vi "PIM Convert 1.1 to 1.2.vi"(0 "PIM 1.1 Test Parameters":T8={"PIM Test Stimulus"={"C1 Pwr dBm"=0.0, "C2 Pwr dBm"=0.0, "Power Units"=enum."dBm", "Meas Type"=enum."Band Edges", "C1 Fixed MHz"=0.0, "C2 Fixed MHz"=0.0, "Swept Freq Step"=0}, "Measure"={"IM Order"=0, "Direction"=0, "Averaging"=1, "ALC ON?"=TRUE, "Peak Hold?"=TRUE, "Peak last N"=1, "Ref Level dBm"=-100.0, "Ref Units"=enum."dBm", "Num Samples"=1, "Sample units"=enum."Sample(s)", "Update Rate (s)"=0.0}, "Display"={"Power Scale"={"yRange_min"=-160, "yRange_max"=-60}, "xRange_span"=0}, "Datasheets"=[]} {"Display"."xRange_span" min=5 step=1; "Display"."Power Scale"."yRange_max" min=-200 max=0 step=1; "Display"."Power Scale"."yRange_min" min=-200 max=0 step=1; "Measure"."Update Rate (s)" min=-200.0 max=0.0 step=0.2 format="%.1f"; "Measure"."Num Samples" min=1 max=5000 step=1; "Measure"."Averaging" items=["None", "Minimum", "Normal", "High", "Maximum"]; "Measure"."Ref Level dBm" min=-200.0 max=0.0 step=0.2 format="%.1f"; "Measure"."Peak last N" min=1 max=5000 step=1; "Measure"."Direction" items=["Reverse", "Forward", "Auxiliary"]; "Measure"."IM Order" items=["3rd", "5th", "7th", "9th", "11th", "13th", "15th", "17th", "19th", "21st", "23rd", "25th", "27th", "29th", "31st", "33rd"]; "PIM Test Stimulus"."C2 Fixed MHz" min=-200.0 max=0.0 step=0.2 format="%.1f"; "PIM Test Stimulus"."C1 Fixed MHz" min=-200.0 max=0.0 step=0.2 format="%.1f"; "PIM Test Stimulus"."Swept Freq Step" items=[".2", ".4", "1.0", "2.0"]}) -> (1 "Datasheets":T7, 2 "PIM 1.2 Test Parameters":T1={"Stimulus"={"C1 Pwr dBm"=0.0, "C2 Pwr dBm"=0.0, "Power Units"=enum."dBm", "Meas Type"=enum."Fixed Pair", "C1 Fixed MHz"=0.0, "C2 Fixed MHz"=0.0, "Swept Freq Step"=0}, "Measure"={"IM Order"=0, "Direction"=0, "Averaging"=0, "ALC ON?"=FALSE, "Peak Hold?"=FALSE, "Peak last N"=0, "Ref Level dBm"=0.0, "Ref Units"=enum."dBm", "Num Samples"=0, "Sample units"=enum."Sample(s)", "Update Rate (s)"=0.0}, "Display"={"Power Scale"={"yRange_min"=0, "yRange_max"=0}, "xRange_span"=0}} {"Stimulus"."C2 Fixed MHz" min=-200.0 max=0.0 step=0.2 format="%.1f"; "Stimulus"."C1 Fixed MHz" min=-200.0 max=0.0 step=0.2 format="%.1f"; "Stimulus"."Swept Freq Step" items=[".2", ".4", "1.0", "2.0"]; "Measure"."IM Order" items=["3rd", "5th", "7th", "9th", "11th", "13th", "15th", "17th", "19th", "21st", "23rd", "25th", "27th", "29th", "31st", "33rd"]; "Measure"."Direction" items=["Reverse", "Forward", "Auxiliary"]; "Measure"."Averaging" items=["None", "Minimum", "Normal", "High", "Maximum"]})   [LabVIEW 2011]
uses:
  TypeDefs/PIM Test Parameters v1.1.ctl
  Test Datasheets v1.0-4.0.ctl
  TypeDefs/PIM Test Parameters v1.2-1.3.ctl
  SI.LIB/PIM.LIB/HW IO/IMOrder.ctl
  SI.LIB/PIM.LIB/HW IO/MeasMode.ctl
  SI.LIB/PIM.LIB/HW IO/HW Averaging.ctl
  TypeDefs/PIM Meas Units.ctl
  TypeDefs/PIM Display Parameters.ctl
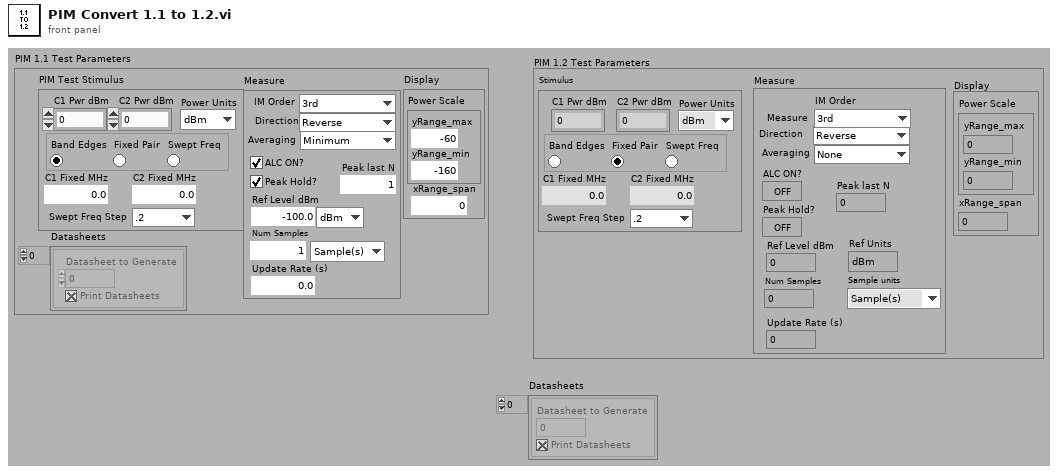
[diagram p1: front panel]
types:
  T1 = typedef "PIM Test Parameters v1.2-1.3.ctl" = cluster{"Stimulus":cluster{"C1 Pwr dBm":dbl, "C2 Pwr dBm":dbl, "Power Units":enum16{"dBm", "Watts"}, "Meas Type":enum32{"Band Edges", "Fixed Pair", "Swept Freq"}, "C1 Fixed MHz":dbl, "C2 Fixed MHz":dbl, "Swept Freq Step":u16}, "Measure":cluster{"IM Order":T2, "Direction":T3, "Averaging":T4, "ALC ON?":bool, "Peak Hold?":bool, "Peak last N":u32, "Ref Level dBm":dbl, "Ref Units":enum16{"dBm", "dBc"}, "Num Samples":u32, "Sample units":T5, "Update Rate (s)":dbl}, "Display":T6}
  T2 = typedef "IMOrder.ctl" = u8
  T3 = typedef "MeasMode.ctl" = u16
  T4 = typedef "HW Averaging.ctl" = u16
  T5 = typedef "PIM Meas Units.ctl" = enum16{"Sample(s)", "Second(s)", "Sweep(s)"}
  T6 = typedef "PIM Display Parameters.ctl" = cluster{"Power Scale":cluster{"yRange_min":i32, "yRange_max":i32}, "xRange_span":u32}
  T7 = typedef "Test Datasheets v1.0-4.0.ctl" = cluster{"Datasheet to Generate":i32, "Print Datasheets":bool}[]
  T8 = typedef "PIM Test Parameters v1.1.ctl" = cluster{"PIM Test Stimulus":cluster{"C1 Pwr dBm":dbl, "C2 Pwr dBm":dbl, "Power Units":enum16{"dBm", "Watts"}, "Meas Type":enum32{"Band Edges", "Fixed Pair", "Swept Freq"}, "C1 Fixed MHz":dbl, "C2 Fixed MHz":dbl, "Swept Freq Step":u16}, "Measure":cluster{"IM Order":u8, "Direction":u16, "Averaging":u16, "ALC ON?":bool, "Peak Hold?":bool, "Peak last N":u32, "Ref Level dBm":dbl, "Ref Units":enum16{"dBm", "dBc"}, "Num Samples":u32, "Sample units":enum16{"Sample(s)", "Second(s)", "Sweep(s)"}, "Update Rate (s)":dbl}, "Display":cluster{"Power Scale":cluster{"yRange_min":i32, "yRange_max":i32}, "xRange_span":u32}, "Datasheets":cluster{"Datasheet to Generate":i32, "Print Datasheets":bool}[]}
  T9 = cluster{"C1 Pwr dBm":dbl, "C2 Pwr dBm":dbl, "Power Units":enum16{"dBm", "Watts"}, "Meas Type":enum32{"Band Edges", "Fixed Pair", "Swept Freq"}, "C1 Fixed MHz":dbl, "C2 Fixed MHz":dbl, "Swept Freq Step":u16}
  T10 = cluster{"IM Order":u8, "Direction":u16, "Averaging":u16, "ALC ON?":bool, "Peak Hold?":bool, "Peak last N":u32, "Ref Level dBm":dbl, "Ref Units":enum16{"dBm", "dBc"}, "Num Samples":u32, "Sample units":enum16{"Sample(s)", "Second(s)", "Sweep(s)"}, "Update Rate (s)":dbl}
  T11 = cluster{"Power Scale":cluster{"yRange_min":i32, "yRange_max":i32}, "xRange_span":u32}
  T12 = cluster{"Datasheet to Generate":i32, "Print Datasheets":bool}[]
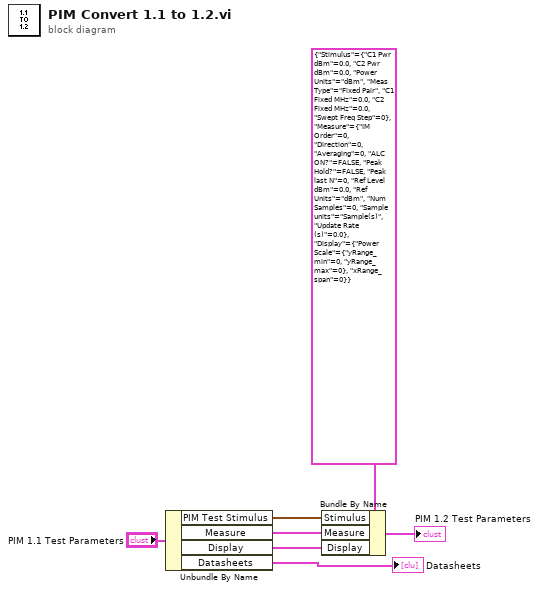
[diagram p0: block diagram]
diagram:
  n1 = Unbundle By Name("PIM 1.1 Test Parameters") -> ("PIM Test Stimulus"=w3:T9, "Measure"=w5:T10, "Display"=w6:T11, "Datasheets"=→"Datasheets":T12)
  n2 = Bundle By Name(cluster=T1 {"Stimulus"={"C1 Pwr dBm"=0.0, "C2 Pwr dBm"=0.0, "Power Units"=enum."dBm", "Meas Type"=enum."Fixed Pair", "C1 Fixed MHz"=0.0, "C2 Fixed MHz"=0.0, "Swept Freq Step"=0}, "Measure"={"IM Order"=0, "Direction"=0, "Averaging"=0, "ALC ON?"=FALSE, "Peak Hold?"=FALSE, "Peak last N"=0, "Ref Level dBm"=0.0, "Ref Units"=enum."dBm", "Num Samples"=0, "Sample units"=enum."Sample(s)", "Update Rate (s)"=0.0}, "Display"={"Power Scale"={"yRange_min"=0, "yRange_max"=0}, "xRange_span"=0}} ("PIM 1.1 Test Parameters"), "Stimulus"=w3, "Measure"=w5, "Display"=w6) -> (→"PIM 1.2 Test Parameters":T1)
